vi "roboRIO v1.0 Shutdown SPI.vi"(8 "error in (no error)":errorcluster, 10 "SPI Channel":T3, 11 "myRIO Ref In":T1) -> (0 "error out":errorcluster, 3 "myRIO Ref Out":T1)   [LabVIEW 2021]
uses:
  <vilib>/myRIO/Common/Instrument Driver Framework/myRIO v1.0/SPI/typedefs/SPI Channels Enum.ctl
  <vilib>/myRIO/Common/Instrument Driver Framework/Utilities/typedefs/myRIO v1.0 Reference.ctl
  <vilib>/myRIO/Common/Instrument Driver Framework/Utilities/typedefs/Generic FPGA Reference.ctl
  <vilib>/myRIO/Common/Instrument Driver Framework/roboRIO v1.0/SPI/typedefs/roboRIO SPI Channels FPGA Reference.ctl
  <vilib>/rvi/errors/niLvFpgaAdjustHostInterfaceError.vi
  <vilib>/rvi/interface/nirviReadWriteControl/nirviReadWriteControl.xnode
  <vilib>/rvi/interface/Simulation/niFpgaSimulationCallBeginRW.vi
  NiFpgaLv.dll
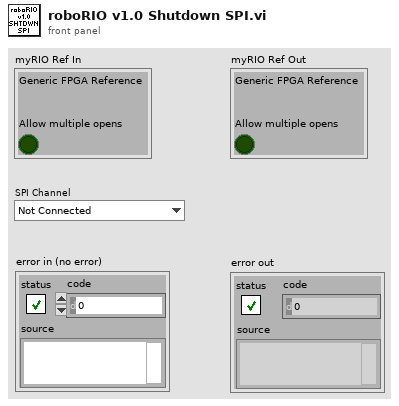
[diagram p1: front panel]
types:
  T1 = typedef "myRIO v1.0 Reference.ctl" = cluster{"Generic FPGA Reference":T2, "Allow multiple opens":bool}
  T2 = typedef "Generic FPGA Reference.ctl" = refnum<k20>
  T3 = typedef "SPI Channels Enum.ctl" = enum16{"Not Connected", "A/SPI", "B/SPI", "SPI/SPI"}
  T4 = typedef "roboRIO SPI Channels FPGA Reference.ctl" = refnum<k20>
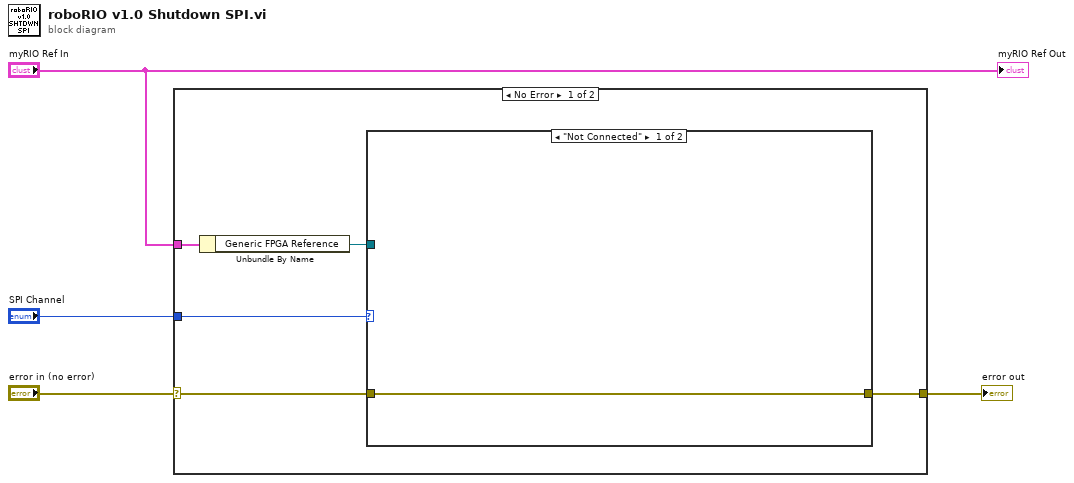
[diagram p0: block diagram]
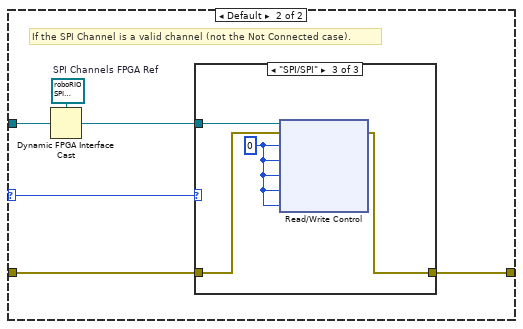
[diagram p2: hidden frame]
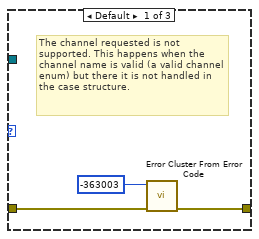
[diagram p3: hidden frame]
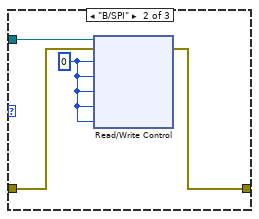
[diagram p4: hidden frame]
diagram:
  n1 = case shown="No Error" "error in (no error)" {
    selector: "error in (no error)" -> [w8 w28]
    tunnel: [w9 w28] -> w4
    tunnel: "myRIO Ref In" -> [w7 _]
    tunnel: "SPI Channel" -> [w6 _]
    frame No Error {
      n2 = Unbundle By Name(w7) -> ("Generic FPGA Reference"=w5:T2)
      n3 = case shown="\"Not Connected\"" w6 {
        selector: w6 -> [_ w11]
        tunnel: [w10 w14] -> w9
        tunnel: w8 -> [w10 w13]
        tunnel: w5 -> [_ w12]
        frame "Not Connected" {
        }
        frame Default {
          w16 = T4 refnum  # SPI Channels FPGA Ref
          # "If the SPI Channel is a valid channel (not the Not Connected case)."
          n4 = Dynamic FPGA Interface Cast(Session In=w16, Type=w12) -> (Session Out=w15:T4)
          n5 = case shown="\"SPI/SPI\"" w11 {
            tunnel: w13 -> [w17 w23 w27]
            tunnel: [w18 w22 w26] -> w14
            tunnel: w15 -> [_ w21 w25]
            frame Default {
              # "The channel requested is not supported. This happens when the channel name is valid (a valid channel enum) but there it is not handled in the case structure."
              n6 = call <vilib>:"Error Cluster From Error Code.vi"("error in (no error)"=w17, "error code (0)"=-363003) -> ("error out"=w18:errorcluster)  [unwired: 7 in]
            }
            frame "B/SPI" {
              w20 = u16 0 ("SPI.A.DATO")
              n7 = xnode "Read/Write Control"("FPGA VI Reference In"=w21, "error in"=w23, "SPI.B.DATO"=w20, "SPI.B.DATI"=w20, "SPI.B.CNFG"=w20, "SPI.B.CNT"=w20, "SPI.B.STAT"=w20) -> ("error out"=w22:errorcluster)  [unwired: 1 out]
            }
            frame "SPI/SPI" {
              w24 = u16 0 ("SPI.A.DATO")
              n8 = xnode "Read/Write Control"("FPGA VI Reference In"=w25, "error in"=w27, "SPI.SPI.DATO"=w24, "SPI.SPI.DATI"=w24, "SPI.SPI.CNFG"=w24, "SPI.SPI.CNT"=w24, "SPI.SPI.STAT"=w24) -> ("error out"=w26:errorcluster)  [unwired: 1 out]
            }
          }
        }
      }
    }
    frame Error {
    }
  }
  "error out" <- w4
  "myRIO Ref Out" <- "myRIO Ref In"
